vi "pAmp_HISTO_GEN.vi"(0 "TCP Network Connection in":refnum<k5>, 2 "COUNTS":u32=100, 3 "CONTINOUS":bool, 4 "ENABLE":bool, 5 "error in (no error)":errorcluster) -> (14 "TCP Network Connection out":refnum<k5>, 16 "STATUS":u32, 19 "error out":errorcluster)   [LabVIEW 2019, in "Histogram.lvlib"]
uses:
  Histogram.lvlib
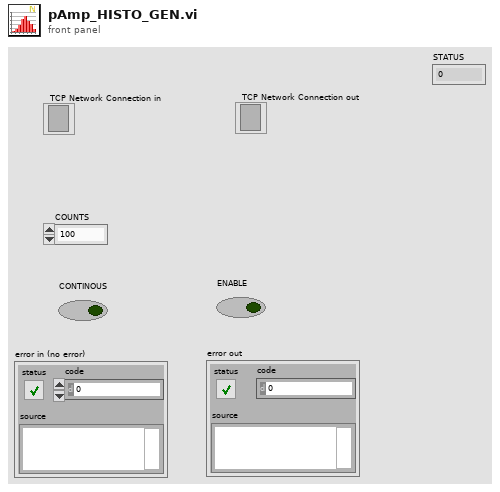
[diagram p1: front panel]
types:
  T1 = enum16{"big-endian, network order", "native, host order", "little-endian"}
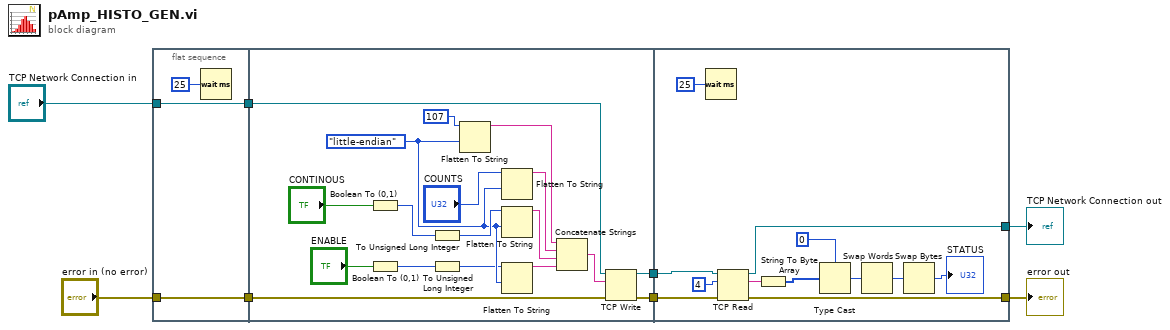
[diagram p0: block diagram]
diagram:
  n1 = flat-sequence {
    tunnel: [w10] -> w4
    tunnel: [w11] -> w3
    tunnel: "error in (no error)" -> [w11]
    tunnel: "TCP Network Connection in" -> [w10]
    tunnel: w4 -> [w29]
    tunnel: w3 -> [w28]
    tunnel: [w27] -> w2
    tunnel: [w26] -> w1
    tunnel: [w38] -> w6
    tunnel: [w39] -> w5
    tunnel: w2 -> [w41]
    tunnel: w1 -> [w40]
    frame #0 {
      n2 = Wait (ms)(milliseconds to wait=u32 25) -> ()  [unwired: 1 out]
    }
    frame #1 {
      w16 = T1."little-endian" ("byte order (0:big-endian, network order)")
      n3 = Boolean To (0,1)(Boolean="CONTINOUS") -> (0, 1=w18:i16)
      n4 = Boolean To (0,1)(Boolean="ENABLE") -> (0, 1=w14:i16)
      n5 = To Unsigned Long Integer(number=w18) -> (unsigned 32bit integer=w17:u32)
      n6 = To Unsigned Long Integer(number=w14) -> (unsigned 32bit integer=w13:u32)
      n7 = Flatten To String(anything=u32 107 ("element"), byte order (0:big-endian, network order)=w16) -> (data string=w23:string)  [unwired: 2 in, 2 out]
      n8 = Flatten To String(anything="COUNTS", byte order (0:big-endian, network order)=w16) -> (data string=w25:string)  [unwired: 2 in, 2 out]
      n9 = Flatten To String(anything=w17, byte order (0:big-endian, network order)=w16) -> (data string=w20:string)  [unwired: 2 in, 2 out]
      n10 = Flatten To String(anything=w13, byte order (0:big-endian, network order)=w16) -> (data string=w12:string)  [unwired: 2 in, 2 out]
      n11 = Concatenate Strings(w23, w25, w20, w12) -> (w22:string)
      n12 = TCP Write(connection ID=w29, data in=w22, error in (no error)=w28) -> (connection ID out=w27:refnum<k5>, error out=w26:errorcluster)  [unwired: 1 in, 1 out]
    }
    frame #2 {
      n13 = Wait (ms)(milliseconds to wait=u32 25) -> ()  [unwired: 1 out]
      n14 = TCP Read(connection ID=w41, bytes to read=4, error in (no error)=w40) -> (connection ID out=w39:refnum<k5>, data out=w35:string, error out=w38:errorcluster)  [unwired: 2 in]
      n15 = String To Byte Array(string=w35) -> (unsigned byte array=w32:u8[])
      n16 = Type Cast(type=u32 0 ("index"), x=w32) -> (*(type *) &x=w34:u32)
      n17 = Swap Words(1:w34) -> (0:w33:u32)
      n18 = Swap Bytes(anything=w33) -> (byte swapped=→"STATUS":u32)
    }
  }
  "error out" <- w6
  "TCP Network Connection out" <- w5
